vi "Ctrl.StyleFont.vi"(8 "error in (no error)":errorcluster, 10 "Font Info":T1, 11 "Ctl Ref in":refnum<vi>) -> (0 "error out":errorcluster, 3 "Ctl Ref out":refnum<vi>)   [LabVIEW 2020]
uses:
  Font Info -- Cluster.ctl
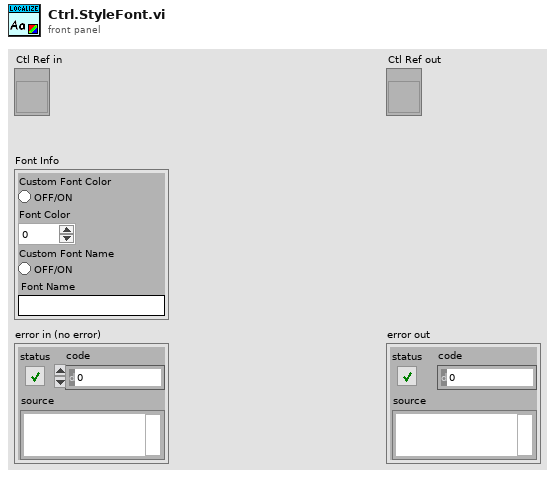
[diagram p1: front panel]
types:
  T1 = typedef "Font Info -- Cluster.ctl" = cluster{"Custom Font Color":bool, "Font Color":u32, "Custom Font Name":bool, "Font Name":string}
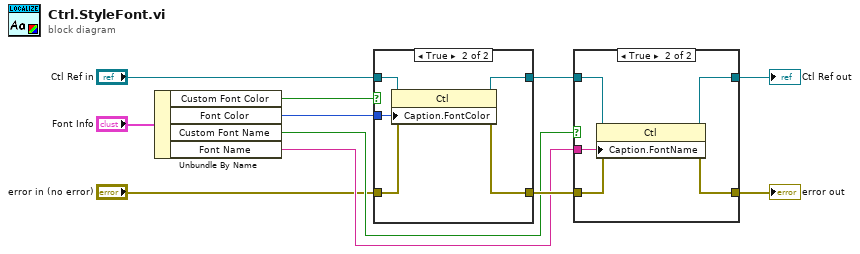
[diagram p0: block diagram]
diagram:
  n1 = Unbundle By Name("Font Info") -> ("Custom Font Color"=w9:bool, "Font Color"=w8:u32, "Custom Font Name"=w4:bool, "Font Name"=w5:string)
  n2 = case shown="True" w9 {
    tunnel: "Ctl Ref in" -> [w13 w18]
    tunnel: w8 -> [_ w17]
    tunnel: [w12 w16] -> w7
    tunnel: [w13 w15] -> w6
    tunnel: "error in (no error)" -> [w12 w14]
    frame False {
    }
    frame True {
      n3 = property class="Ctl"(reference=w18, error in=w14, "Caption.FontColor"=w17) -> (reference out=w15:refnum<vi>, error out=w16:errorcluster)
    }
  }
  n4 = case shown="True" w4 {
    tunnel: w7 -> [w19 w25]
    tunnel: [w20 w23] -> w2
    tunnel: w6 -> [w20 w24]
    tunnel: w5 -> [_ w22]
    tunnel: [w19 w21] -> w1
    frame False {
    }
    frame True {
      n5 = property class="Ctl"(reference=w24, error in=w25, "Caption.FontName"=w22) -> (reference out=w23:refnum<vi>, error out=w21:errorcluster)
    }
  }
  "Ctl Ref out" <- w2
  "error out" <- w1
